vi "CSMKVMap-Read.vi"(8 "Error in":errorcluster caption="Error in (no error)", 10 "default value (empty variant)":variant, 11 "name":string) -> (0 "Error out":errorcluster, 3 "value":variant)   [LabVIEW 2017, in "Communicable State Machine.lvlib"]
uses:
  Communicable State Machine.lvlib
  _Support/ChangeFlag/ChangeFlag-Read.vi
  _Support/ChangeFlag/ChangeFlagDB.vi
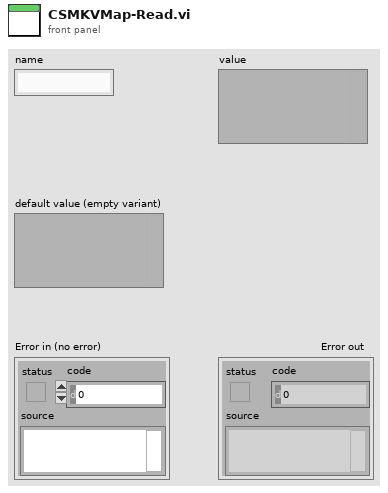
[diagram p1: front panel]
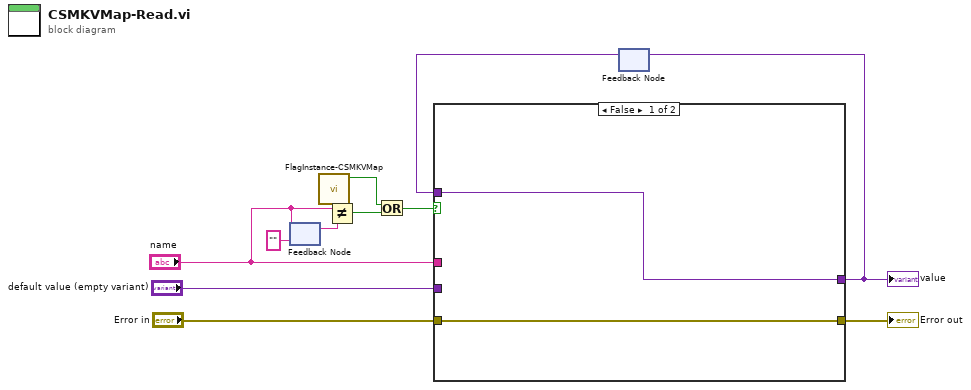
[diagram p0: block diagram]
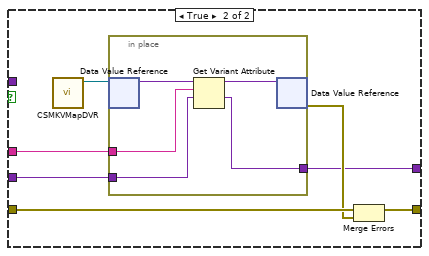
[diagram p2: hidden frame]
diagram:
  n1 = feedback #1("" ("name")) -> (w8:string)
  n2 = feedback-in #1("name") -> ()
  n3 = call "FlagInstance-CSMKVMap.vi"() -> ("Changed"=w4:bool)  [unwired: 10 in, 1 out]
  n4 = Not Equal?(x="name", y=w8) -> (x != y?=w5:bool)
  n5 = Or(x=w4, y=w5) -> (x .or. y?=w3:bool)
  n6 = feedback #2() -> (w1:variant)  [unwired: 1 in]
  n7 = case shown="False" w3 {
    tunnel: "name" -> [_ w19]
    tunnel: "Error in" -> [w13 w18]
    tunnel: [w13 w17] -> w10
    tunnel: "default value (empty variant)" -> [_ w15]
    tunnel: [w12 w14] -> w2
    tunnel: w1 -> [w12 _]
    frame False {
    }
    frame True {
      n8 = call "CSMKVMapDVR.vi"() -> ("KVMapDVR"=w20:refnum<data-value>)  [unwired: 11 in]
      n9 = in-place {
        in-place-border: w19 -> [w23]
        in-place-border: w15 -> [w22]
        in-place-border: [w21] -> w14
        n10 = in-place-dvr #3(w20) -> (w25:variant)  [unwired: 1 out]
        n11 = Get Variant Attribute(Variant=w25, name=w23, default value (empty Variant)=w22) -> (duplicate Variant=w24:variant, value=w21:variant)  [unwired: 1 in, 2 out]
        n12 = in-place-dvr #3(w24) -> (w16:errorcluster)  [unwired: 1 out]
      }
      n13 = Merge Errors(w18, w16) -> (w17:errorcluster)
    }
  }
  "Error out" <- w10
  "value" <- w2
  n14 = feedback-in #2(w2) -> ()
